vi "MarlinSerial – GetTemps.vi"(0 "VISA Refnum in":refnum<visa-resource-name>, 1 "Poll temps":bool=TRUE, 5 "Poll temps interval":i32, 7 "Loop wait ( ms )":i32, 9 "Loop iteration":i32, 11 "error in (no error)":errorcluster) -> (3 "read buffer":string, 4 "VISA Refnum out":refnum<visa-resource-name>, 6 "Grabbed float":dbl, 8 "Grabbed float 2":dbl, 15 "error out":errorcluster)   [LabVIEW 2020]
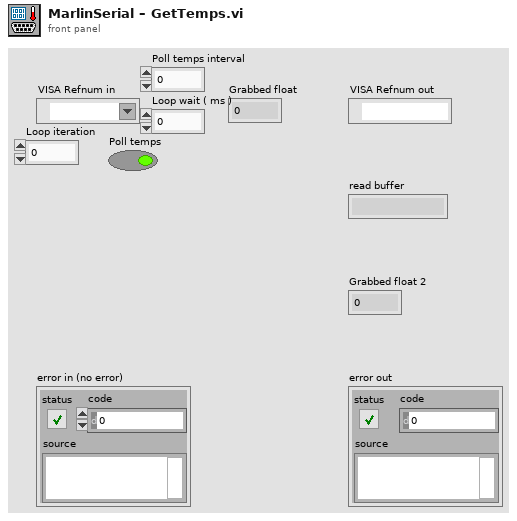
[diagram p1: front panel]
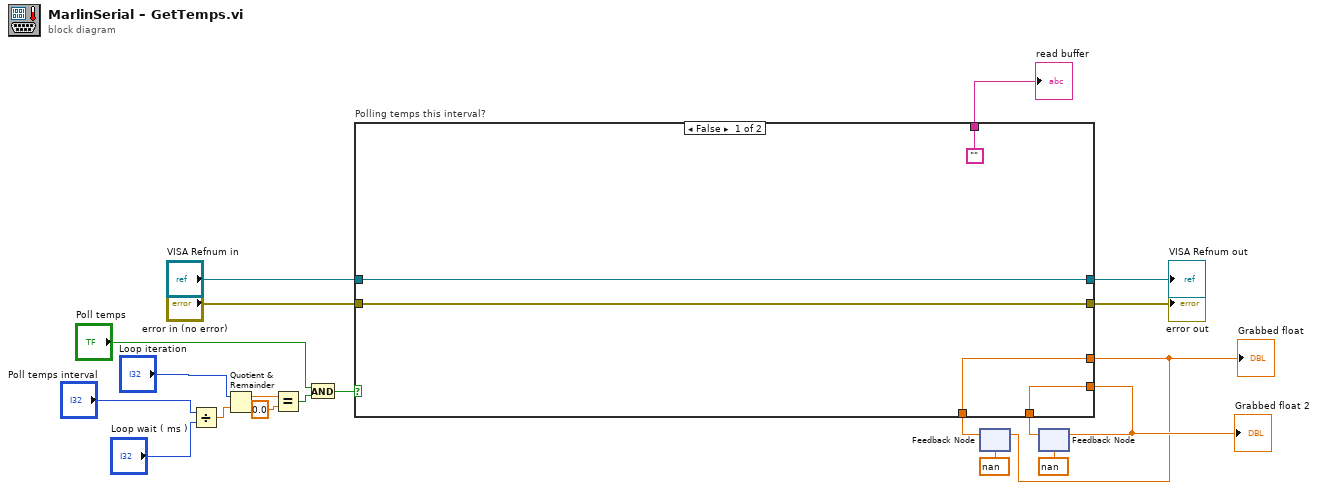
[diagram p0: block diagram]
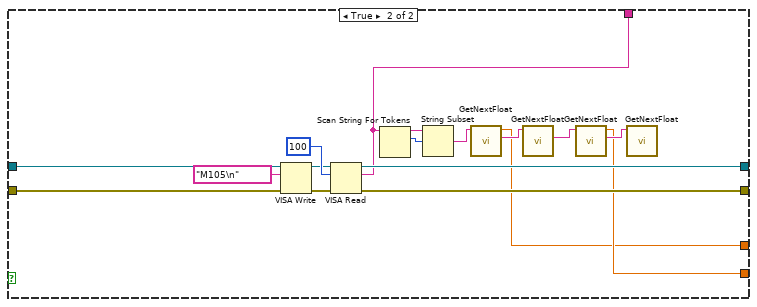
[diagram p2: hidden frame]
diagram:
  n1 = Divide(x="Poll temps interval", y="Loop wait ( ms )") -> (x/y=w16:dbl)
  n2 = Quotient & Remainder(x="Loop iteration", y=w16) -> (x-y*floor(x/y)=w15:dbl)  [unwired: 1 out]
  n3 = Equal?(x=w15, y=0.0) -> (x = y?=w13:bool)
  n4 = And(x="Poll temps", y=w13) -> (x .and. y?=w12:bool)
  n5 = feedback #1(nan) -> (w2:dbl)
  n6 = feedback #2(nan) -> (w3:dbl)
  n7 = case "Polling temps this interval?" shown="False" w12 {
    tunnel: "VISA Refnum in" -> [w22 w34]
    tunnel: [w22 w31] -> w19
    tunnel: "error in (no error)" -> [w23 w30]
    tunnel: [w23 w29] -> w17
    tunnel: [w25 w28] -> w5
    tunnel: [w24 w27] -> w4
    tunnel: w3 -> [w25 _]
    tunnel: w2 -> [w24 _]
    tunnel: ["" w26] -> w1
    frame False {
    }
    frame True {
      n8 = VISA Write(VISA resource name=w34, write buffer="M105\n", error in (no error)=w30) -> (VISA resource name out=w32:refnum<visa-resource-name>, error out=w33:errorcluster)  [unwired: 1 out]
      n9 = VISA Read(VISA resource name=w32, byte count=u32 100, error in (no error)=w33) -> (VISA resource name out=w31:refnum<visa-resource-name>, read buffer=w26:string, error out=w29:errorcluster)  [unwired: 1 out]
      n10 = Scan String For Tokens(9:w26) -> (2:w40:i32, 3:w39:string)  [unwired: 5 in, 2 out]
      n11 = String Subset(string=w39, offset (0)=w40) -> (substring=w41:string)  [unwired: 1 in]
      n12 = call "GetNextFloat.vi"("read buffer in"=w41) -> ("remaining string"=w36:string, "Grabbed float"=w27:dbl)  [unwired: 9 in]
      n13 = call "GetNextFloat.vi"("read buffer in"=w36) -> ("remaining string"=w37:string)  [unwired: 9 in, 1 out]
      n14 = call "GetNextFloat.vi"("read buffer in"=w37) -> ("remaining string"=w38:string, "Grabbed float"=w28:dbl)  [unwired: 9 in]
      n15 = call "GetNextFloat.vi"("read buffer in"=w38) -> ()  [unwired: 9 in, 2 out]
    }
  }
  "read buffer" <- w1
  "VISA Refnum out" <- w19
  "error out" <- w17
  "Grabbed float 2" <- w5
  "Grabbed float" <- w4
  n16 = feedback-in #1(w4) -> ()
  n17 = feedback-in #2(w5) -> ()
